vi "sv_Check Data Valid (N Ch) [Weighting].vi"(6 "reset (in)":bool, 8 "error in (no error)":errorcluster, 9 "weighting":T1 items=["Linear", "A-weighting", "B-weighting", "C-weighting", "ITU-R 468-4", "Dolby", "CCITT", "C-message", "Wb", "Wc", "Wd", "We", "Wf", "Wh", "Wj", "Wk", "Wm", "AES17 20 kHz lowpass", "AES17 40 kHz lowpass", "AES17 20 kHz highpass", "AES17 40 kHz highpass"], 11 "scaled signal [in]":waveform(dbl)[](array[waveform])) -> (0 "error out":errorcluster, 1 "weighting":T1 items=["Linear", "A-weighting", "B-weighting", "C-weighting", "ITU-R 468-4", "Dolby", "CCITT", "C-message", "Wb", "Wc", "Wd", "We", "Wf", "Wh", "Wj", "Wk", "Wm", "AES17 20 kHz lowpass", "AES17 40 kHz lowpass", "AES17 20 kHz highpass", "AES17 40 kHz highpass"], 3 "scaled signal [out]":waveform(dbl)[](array[waveform]), 4 "reset (out)":bool)   [LabVIEW 2017]
uses:
  <vilib>/addons/_NISVFA/_Shared subVIs/Controls/svc_Weighting Filter Text Ring.ctl
  <vilib>/addons/_NISVFA/_Shared subVIs/Common/svc_Check for Waveform Parameter Continuity (no state).vi
  <vilib>/addons/_NISVFA/_Shared subVIs/Common/svc_Get SV Channel Info.vi
  <vilib>/addons/_NISVFA/_Shared subVIs/Common/svc_Engineering Units to Unit Label.vi
  <vilib>/addons/_NISVFA/_Shared subVIs/Common/svc_Unit Label to Engineering Units.vi
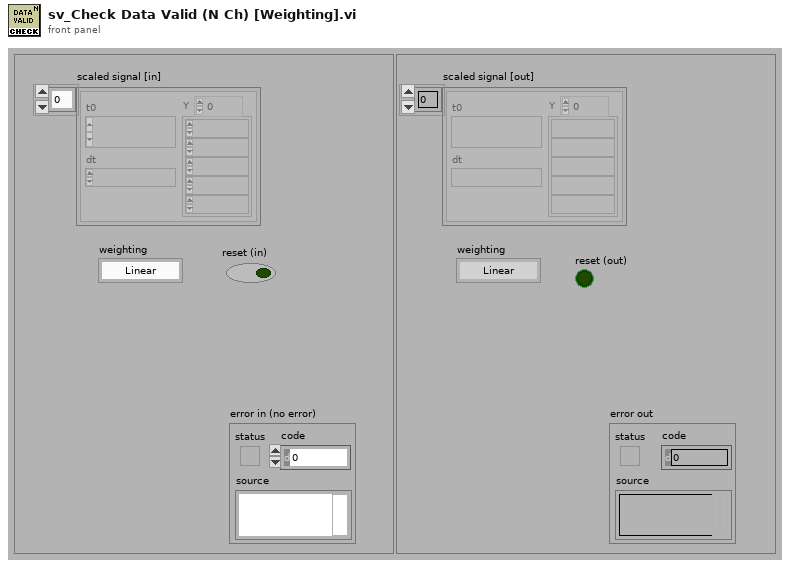
[diagram p1: front panel]
types:
  T1 = typedef "svc_Weighting Filter Text Ring.ctl" = u16
  T2 = cluster{"dt equal":bool, "array length equal":bool, "number channels change":bool}
  T3 = cluster{"dt":bool, "t0 continuity":bool, "array length":bool, "channel info":bool, "name":bool}
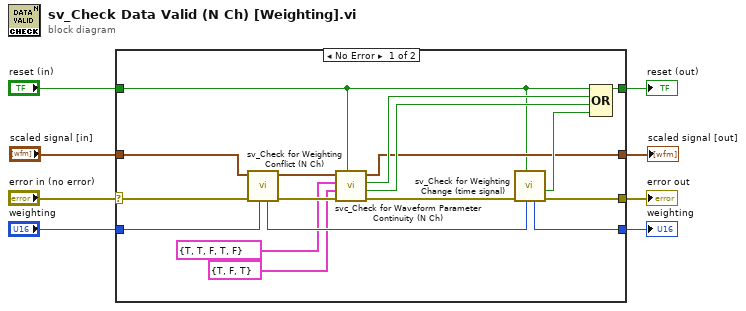
[diagram p0: block diagram]
diagram:
  n1 = case shown="No Error" "error in (no error)" {
    selector: "error in (no error)" -> [w23 w28]
    tunnel: [w21 w28] -> w8
    tunnel: "scaled signal [in]" -> [w14 w26]
    tunnel: "reset (in)" -> [w13 w29]
    tunnel: [w24 w29] -> w6
    tunnel: "weighting" -> [w25 w27]
    tunnel: [w20 w27] -> w3
    tunnel: [w15 w26] -> w1
    frame No Error {
      n2 = call <vilib>:"sv_Check for Weighting Conflict (N Ch).vi"("weighting"=w25, "error in (no error)"=w23, "scaled signals"=w14) -> ("error out"=w17:errorcluster, "dup scaled signals"=w16:waveform(dbl)[], "weighting"=w11:T1)  [unwired: 6 in]
      n3 = call <vilib>:"svc_Check for Waveform Parameter Continuity (N Ch).vi"("restart averaging (F)"=w13, "error in (no error)"=w17, "checks for multichannel parameters"=T2 {"dt equal"=TRUE, "array length equal"=FALSE, "number channels change"=TRUE}, "checks for channel parameter change"=T3 {"dt"=TRUE, "t0 continuity"=TRUE, "array length"=FALSE, "channel info"=TRUE, "name"=FALSE}, "scaled signal(s)"=w16) -> ("error out"=w12:errorcluster, "multichannel parameter changed"=w18:bool, "waveform parameter changed"=w19:bool, "dup scaled signal(s)"=w15:waveform(dbl)[])  [unwired: 3 out]
      n4 = call <vilib>:"sv_Check for Weighting Change (time signal).vi"("weighting"=w11, "reset (in)"=w13, "error in (no error)"=w12) -> ("error out"=w21:errorcluster, "weighting has changed"=w22:bool, "dup weighting"=w20:T1)  [unwired: 6 in]
      n5 = Compound Arithmetic op=OR(w13, w19, w18, w22) -> (w24:bool)
    }
    frame Error {
    }
  }
  "scaled signal [out]" <- w1
  "error out" <- w8
  "reset (out)" <- w6
  "weighting" <- w3
